vi "Cannon GetSensors.vi"(1 "Cannon Global Data In":T2) -> (0 "Cannon Global Data Out":T2)   [LabVIEW 2013]
uses:
  <vilib>/Rock Robotics/WPI/Solenoid/WPI_SolenoidValue.ctl
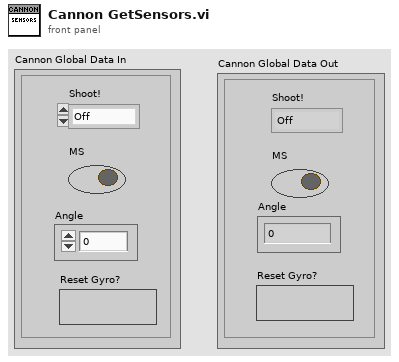
[diagram p1: front panel]
types:
  T1 = typedef "WPI_SolenoidValue.ctl" = enum16{"Off", "On", "Forward", "Reverse"}
  T2 = cluster{"MS":bool, "Shoot!":T1, "Angle":dbl, "Reset Gyro?":bool}
  T3 = typedef "WPI_AnalogChannelDevRef.ctl" = cluster{"DevStatus":errorcluster, "Analog Module":T4, "Analog Channel":T5}
  T4 = typedef "FPGA_TypedefAnalogModule.ctl" = enum16{"Analog Module 1", "Analog Module 2"}
  T5 = typedef "FPGA_AIChannel.ctl" = enum8{"AI 1", "AI 2", "AI 3", "AI 4", "AI 5", "AI 6", "AI 7", "AI 8", "Invalid"}
  T6 = typedef "WPI_GyroDevRef.ctl" = cluster{"DevStatus":errorcluster, "Analog Module":T4, "Analog Channel":T5, "Offset":dbl, "Gain (VoltsPerDegree/Second)":dbl}
  T7 = typedef "WPI_DigitalInputDevRef.ctl" = cluster{"DevStatus":errorcluster, "DIO Channel":T8, "Digital Module":T9}
  T8 = typedef "FPGA_DIOChannel.ctl" = enum8{"DIO 1", "DIO 2", "DIO 3", "DIO 4", "DIO 5", "DIO 6", "DIO 7", "DIO 8", "DIO 9", "DIO 10", "DIO 11", "DIO 12", "DIO 13", "DIO 14", "Invalid"}
  T9 = typedef "FPGA_TypedefDigitalModule.ctl" = enum16{"Digital Module 1", "Digital Module 2"}
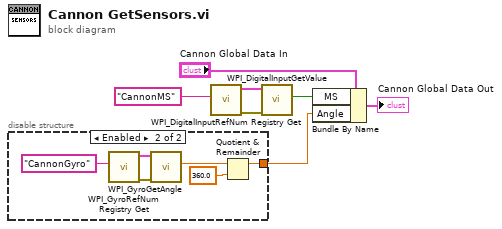
[diagram p0: block diagram]
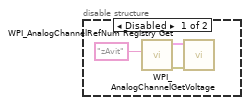
[diagram p2: hidden frame]
diagram:
  n1 = disable-structure shown="Enabled" {
    disable-tunnel: [_ w12] -> w5
    frame Disabled {
      n2 = call <vilib>:"WPI_AnalogChannelRefNum Registry Get.vi"("refnum name"="zAvit") -> ("error out"=w11:errorcluster, "AIDeviceRef"=w10:T3)  [unwired: 9 in]
      n3 = call <vilib>:"WPI_AnalogChannelGetVoltage.vi"("error in (no error)"=w11, "AIDeviceRef"=w10) -> ("Voltage"=w8:dbl)  [unwired: 7 in, 2 out]
    }
    frame Enabled {
      n4 = call "WPI_GyroRefNum Registry Get.vi"("refnum name"="CannonGyro") -> ("error out"=w17:errorcluster, "GyroDevRef"=w16:T6)  [unwired: 9 in]
      n5 = call "WPI_GyroGetAngle.vi"("error in (no error)"=w17, "GyroDevRef"=w16) -> ("Angle"=w15:dbl)  [unwired: 6 in, 3 out]
      n6 = Quotient & Remainder(x=w15, y=360.0) -> (x-y*floor(x/y)=w12:dbl)  [unwired: 1 out]
    }
  }
  n7 = call <vilib>:"WPI_DigitalInputRefNum Registry Get.vi"("refnum name"="CannonMS") -> ("error out"=w3:errorcluster, "DigitalInputDevRef"=w4:T7)  [unwired: 9 in]
  n8 = call <vilib>:"WPI_DigitalInputGetValue.vi"("error in (no error)"=w3, "DigitalInputDevRef"=w4) -> ("Value"=w1:bool)  [unwired: 7 in, 2 out]
  n9 = Bundle By Name(cluster="Cannon Global Data In", "MS"=w1, "Angle"=w5) -> (→"Cannon Global Data Out":T2)
